vi "initStatus.vi"(0 "VisaCluster":T8, 5 "Array 2":string[](array[string]), 7 "Temp_Unit":T4, 11 "error in (no error)":errorcluster) -> (4 "VisaCluster  2":T8, 6 "Array":string[](array[string]), 8 "Control":T6 {"Lower"."Numeric" format="%#_4f"; "Set_Rel"."Numeric" format="%#_4f"; "UPPER"."Numeric" format="%#_4f"}, 10 "Display":T7, 15 "error out":errorcluster)   [LabVIEW 2014, in "FH 55.lvlib"]
doc: "Dieses VI liest alle Parameter aus dem Gerät aus\n\nThis VI reads all parameters from the device"
uses:
  FH 55.lvlib
  TypeDef/Temp_Unit.ctl
  TypeDef/VisaCluster.ctl
  TypeDef/Range.ctl
  TypeDef/Unit2.ctl
  TypeDef/Unit.ctl
  TypeDef/Max.ctl
panel:
  in  "Control 2":T6 {"Lower"."Numeric" format="%#_4f"; "Set_Rel"."Numeric" format="%#_4f"; "UPPER"."Numeric" format="%#_4f"}
  in  "Display 2":T7
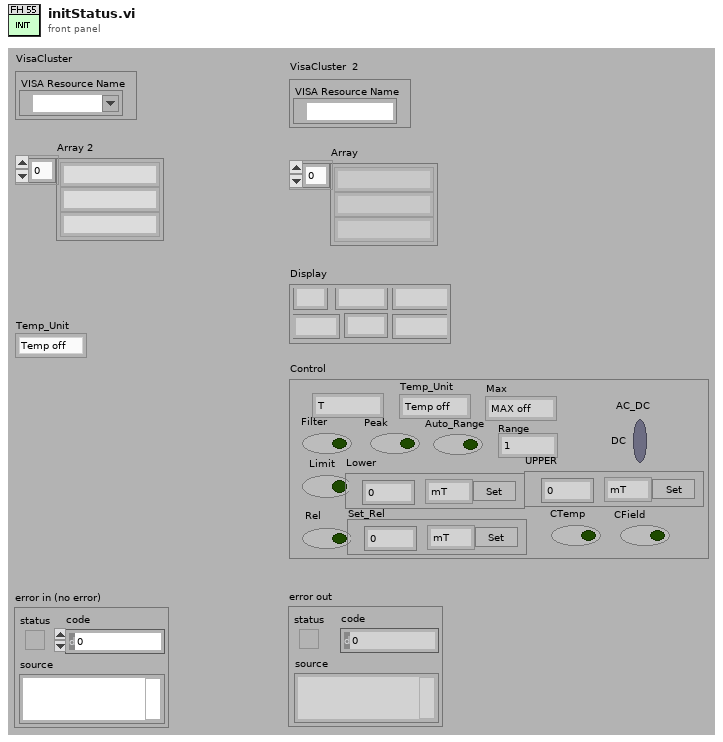
[diagram p1: front panel]
types:
  T1 = typedef "FH 55.lvlib/Range.ctl" = enum16{"1", "2", "3", "4", "5", "6", "7"}
  T2 = typedef "FH 55.lvlib/Unit2.ctl" = enum16{"mT", "G", "kA/m"}
  T3 = typedef "FH 55.lvlib/Unit.ctl" = enum16{"T", "G", "A/m"}
  T4 = typedef "FH 55.lvlib/Temp_Unit.ctl" = enum16{"Temp off", "Celsius", "Fahrenheit"}
  T5 = typedef "FH 55.lvlib/Max.ctl" = enum16{"MAX off", "Show MAX", "MAX/MIN"}
  T6 = cluster{" Peak":bool, " Limit":bool, " Filter":bool, " Auto_Range":bool, " Rel":bool, "AC_DC ":bool, "Range":T1, " CField":bool, " CTemp":bool, "UPPER":cluster{"Numeric":dbl, "Cancel Button":bool, "Unit":T2}, "Set_Rel":cluster{"Numeric":dbl, "Cancel Button":bool, "Unit":T2}, "Unit":T3, "Temp_Unit":T4, "Max":T5, "Lower":cluster{"Numeric":dbl, "Cancel Button":bool, "Unit":T2}}
  T7 = cluster{"AC/DC":string, "Auto":string, "Filter":string, "Range":string, "Rel":string, "Peak":string}
  T8 = typedef "FH 55.lvlib/VisaCluster.ctl" = cluster{"VISA Resource Name":refnum<visa-resource-name>}
  T9 = cluster{"Peak":bool, "Limit":bool, "Filter":bool, "Auto_Range":bool, "Rel":bool, "AC_DC":bool, "Range":T1, "CField":bool, "CTemp":bool, "UPPER":cluster{"Numeric":dbl, "Cancel Button":bool, "Unit":T2}, "Set_Rel":cluster{"Numeric":dbl, "Cancel Button":bool, "Unit":T2}, "Unit":T3, "Temp_Unit":T4, "Max":T5, "Lower":cluster{"Numeric":dbl, "Cancel Button":bool, "Unit":T2}}
  T10 = cluster{"Numeric":dbl, "Cancel Button":bool, "Unit":T2}
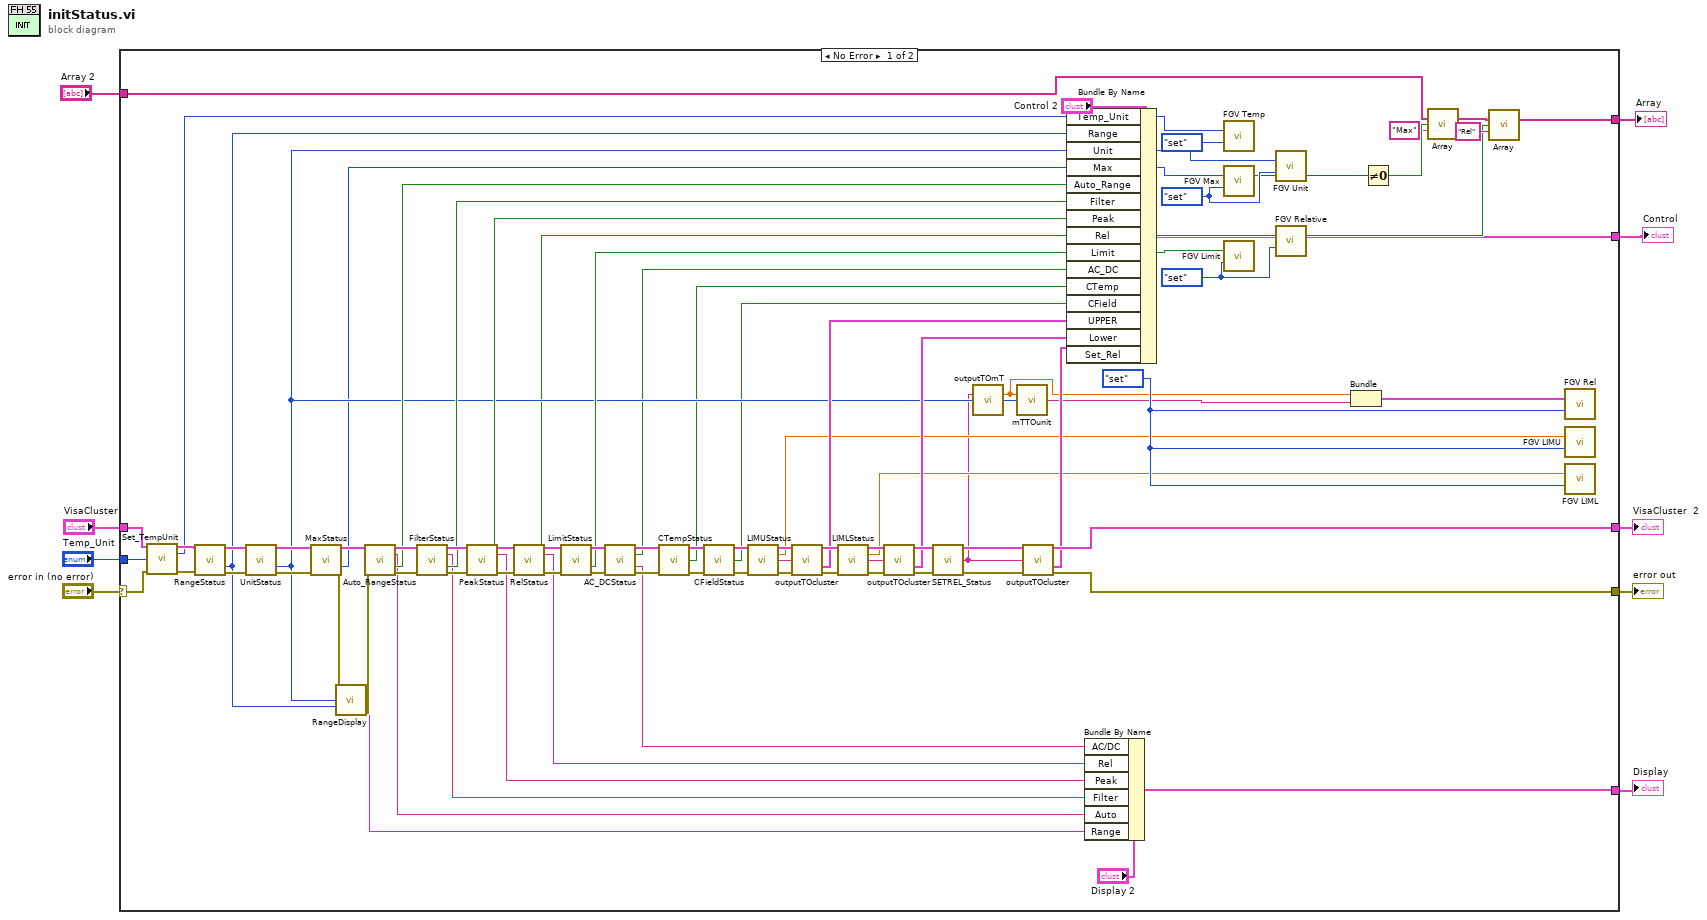
[diagram p0: block diagram]
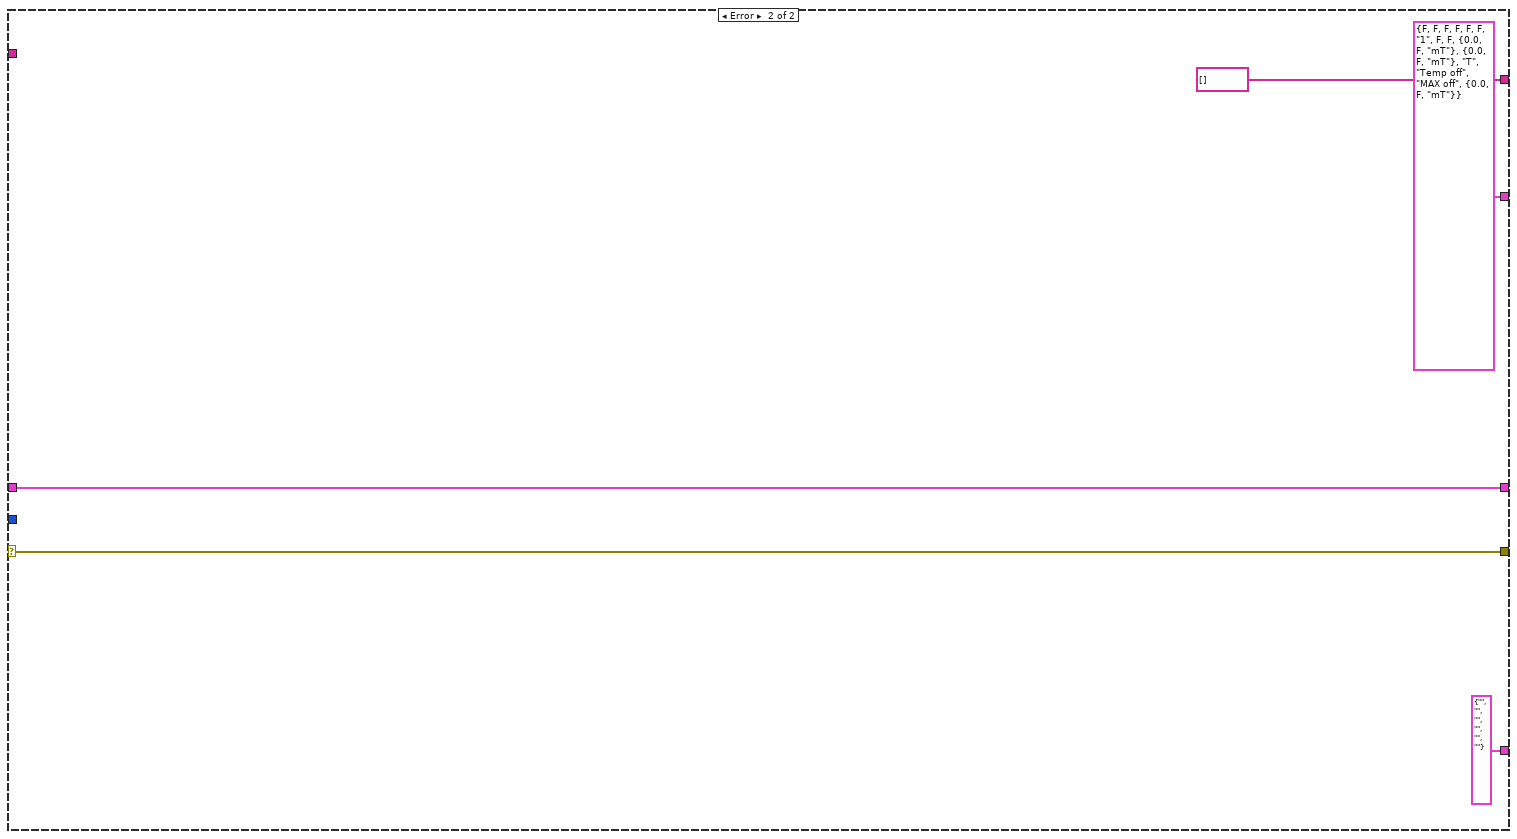
[diagram p2: hidden frame]
diagram:
  n1 = case shown="No Error" "error in (no error)" {
    selector: "error in (no error)" -> [w48 w92]
    tunnel: "Temp_Unit" -> [w88 _]
    tunnel: "VisaCluster" -> [w62 w93]
    tunnel: [w50 w93] -> w6
    tunnel: [w49 w92] -> w5
    tunnel: [w23 T9 {"Peak"=FALSE, "Limit"=FALSE, "Filter"=FALSE, "Auto_Range"=FALSE, "Rel"=FALSE, "AC_DC"=FALSE, "Range"=enum."1", "CField"=FALSE, "CTemp"=FALSE, "UPPER"={"Numeric"=0.0, "Cancel Button"=FALSE, "Unit"=enum."mT"}, "Set_Rel"={"Numeric"=0.0, "Cancel Button"=FALSE, "Unit"=enum."mT"}, "Unit"=enum."T", "Temp_Unit"=enum."Temp off", "Max"=enum."MAX off", "Lower"={"Numeric"=0.0, "Cancel Button"=FALSE, "Unit"=enum."mT"}} ("Control 2")] -> w1
    tunnel: [w42 T7 {"AC/DC"="", "Auto"="", "Filter"="", "Range"="", "Rel"="", "Peak"=""} ("Display 2")] -> w4
    tunnel: "Array 2" -> [w26 _]
    tunnel: [w31 string[] [] ("Array")] -> w2
    frame No Error {
      w19 = enum16{"set", "get"}."set" ("action")
      w34 = enum16{"set", "get"}."set" ("action")
      w36 = enum16{"set", "get"}."set" ("action")
      n2 = call "Set_TempUnit.vi"("VisaCluster"=w62, "Temp_Unit"=w88, "error in (no error)"=w48) -> ("VisaCluster"=w64:T8, "Temp_Unit"=w33:T4, "error out"=w63:errorcluster)  [unwired: 9 in, 1 out]
      n3 = call "RangeStatus.vi"("VisaCluster"=w64, "error in (no error)"=w63) -> ("VisaCluster"=w72:T8, "Range"=w56:T1, "error out"=w70:errorcluster)  [unwired: 10 in, 1 out]
      n4 = call "UnitStatus.vi"("VisaCluster"=w72, "error in (no error)"=w70) -> ("VisaCluster"=w71:T8, "Unit"=w37:T3, "error out"=w69:errorcluster)  [unwired: 10 in, 1 out]
      n5 = call "MaxStatus.vi"("VisaCluster"=w71, "error in (no error)"=w69) -> ("VisaCluster"=w77:T8, "Max"=w30:T5, "error out"=w58:errorcluster)  [unwired: 10 in, 1 out]
      n6 = call "RangeDisplay.vi"("Unit"=w37, "Range"=w56, "error in (no error)"=w58) -> ("Display"=w51:string, "error out"=w57:errorcluster)  [unwired: 10 in, 1 out]
      n7 = call "Auto_RangeStatus.vi"("VisaCluster"=w77, "error in (no error)"=w57) -> ("VisaCluster"=w87:T8, "Display"=w52:string, "Auto_Range"=w61:bool, "error out"=w82:errorcluster)  [unwired: 9 in, 1 out]
      n8 = call "FilterStatus.vi"("VisaCluster"=w87, "error in (no error)"=w82) -> ("VisaCluster"=w86:T8, "Display"=w53:string, "Filter"=w60:bool, "error out"=w81:errorcluster)  [unwired: 9 in, 1 out]
      n9 = call "PeakStatus.vi"("VisaCluster"=w86, "error in (no error)"=w81) -> ("VisaCluster"=w85:T8, "Display"=w54:string, "Peak"=w59:bool, "error out"=w80:errorcluster)  [unwired: 9 in, 1 out]
      n10 = call "RelStatus.vi"("VisaCluster"=w85, "error in (no error)"=w80) -> ("VisaCluster"=w84:T8, "Display"=w55:string, "Rel"=w25:bool, "error out"=w79:errorcluster)  [unwired: 9 in, 1 out]
      n11 = call "LimitStatus.vi"("VisaCluster"=w84, "error in (no error)"=w79) -> ("VisaCluster"=w83:T8, "Limit"=w44:bool, "error out"=w78:errorcluster)  [unwired: 10 in, 1 out]
      n12 = call "AC_DCStatus.vi"("VisaCluster"=w83, "error in (no error)"=w78) -> ("VisaCluster"=w76:T8, "AC_DC"=w11:bool, "Display"=w10:string, "error out"=w74:errorcluster)  [unwired: 9 in, 1 out]
      n13 = call "CTempStatus.vi"("VisaCluster"=w76, "error in (no error)"=w74) -> ("VisaCluster"=w75:T8, "CTemp"=w13:bool, "error out"=w73:errorcluster)  [unwired: 10 in, 1 out]
      n14 = call "CFieldStatus.vi"("VisaCluster"=w75, "error in (no error)"=w73) -> ("VisaCluster"=w67:T8, "CField"=w12:bool, "error out"=w68:errorcluster)  [unwired: 10 in, 1 out]
      n15 = call "LIMUStatus.vi"("VisaCluster"=w67, "error in (no error)"=w68) -> ("VisaCluster"=w66:T8, "Numeric"=w18:dbl, "Message Out"=w17:string, "error out"=w41:errorcluster)  [unwired: 10 in]
      n16 = call "outputTOcluster.vi"("Input"=w17, "error in (no error)"=w41) -> ("Set_lower"=w47:T10, "error out"=w40:errorcluster)  [unwired: 11 in, 1 out]
      n17 = call "LIMLStatus.vi"("VisaCluster"=w66, "error in (no error)"=w40) -> ("VisaCluster"=w65:T8, "Numeric"=w15:dbl, "Message Out"=w16:string, "error out"=w39:errorcluster)  [unwired: 10 in]
      n18 = call "outputTOcluster.vi"("Input"=w16, "error in (no error)"=w39) -> ("Set_lower"=w46:T10, "error out"=w38:errorcluster)  [unwired: 11 in, 1 out]
      n19 = call "SETREL_Status.vi"("VisaCluster"=w65, "error in (no error)"=w38) -> ("VisaCluster"=w50:T8, "Answer"=w14:string, "error out"=w49:errorcluster)  [unwired: 10 in, 1 out]
      n20 = call "outputTOmT.vi"("Input"=w14) -> ("Numeric"=w22:dbl)  [unwired: 13 in, 1 out]
      n21 = call "mTTOunit.vi"("Numeric"=w22, "Unit"=w37) -> ("Display"=w21:string)  [unwired: 11 in, 2 out]
      n22 = call "outputTOcluster.vi"("Input"=w14) -> ("Set_lower"=w45:T10)  [unwired: 12 in, 2 out]
      n23 = Bundle By Name(cluster="Control 2", "Temp_Unit"=w33, "Range"=w56, "Unit"=w37, "Max"=w30, "Auto_Range"=w61, "Filter"=w60, "Peak"=w59, "Rel"=w25, "Limit"=w44, "AC_DC"=w11, "CTemp"=w13, "CField"=w12, "UPPER"=w47, "Lower"=w46, "Set_Rel"=w45) -> (w23:T6)
      n24 = Bundle By Name(cluster="Display 2", "AC/DC"=w10, "Rel"=w55, "Peak"=w54, "Filter"=w53, "Auto"=w52, "Range"=w51) -> (w42:T7)
      n25 = call "FGV Temp.vi"("Temp_Unit"=w33, "action"=enum16{"set", "get"}."set") -> ()  [unwired: 13 in, 1 out]
      n26 = call "FGV Max.vi"("Max"=w30, "action"=w34) -> ()  [unwired: 13 in, 1 out]
      n27 = call "FGV Limit.vi"("Limit"=w44, "action"=w19) -> ()  [unwired: 13 in, 1 out]
      n28 = call "FGV Unit.vi"("Unit"=w37, "action"=w34) -> ()  [unwired: 13 in, 1 out]
      n29 = call "FGV Relative.vi"("Rel"=w25, "action"=w19) -> ()  [unwired: 13 in, 1 out]
      n30 = Bundle("Numeric"=w22, "Display"=w21) -> (w20:cluster{"Numeric":dbl, "Display":string})  [unwired: 1 in]
      n31 = Not Equal To 0?(x=w30) -> (x != 0?=w29:bool)
      n32 = call "Array.vi"("Array"=w26, "Boolean"=w29, "String"="Max") -> ("Array"=w32:string[])  [unwired: 12 in]
      n33 = call "Array.vi"("Array"=w32, "Boolean"=w25, "String"="Rel") -> ("Array"=w31:string[])  [unwired: 12 in]
      n34 = call "FGV Rel.vi"("Extrem_Value"=w20, "action"=w36) -> ()  [unwired: 12 in, 2 out]
      n35 = call "FGV LIMU.vi"("Numeric"=w18, "action"=w36) -> ()  [unwired: 13 in, 1 out]
      n36 = call "FGV LIML.vi"("Numeric"=w15, "action"=w36) -> ()  [unwired: 13 in, 1 out]
    }
    frame Error {
    }
  }
  "error out" <- w5
  "VisaCluster  2" <- w6
  "Display" <- w4
  "Array" <- w2
  "Control" <- w1
